vi "EGE_Query.vi"(0 "System no.":i32=1 min=1 max=4 step=1, 2 "Axes to query":string[](array[string]), 3 "All axes?":bool, 4 "Axis identifier?":bool=TRUE, 5 "error in":errorcluster) -> (14 "Electronic gearing mode":bool[](array[boolean]), 19 "error out":errorcluster)   [LabVIEW 2020]
doc: "Returns electronic gearing mode of queried axes.\n\nC-843, C-848, C-880: If All axes = TRUE, then Axis identifier can be FALSE."
panel:
  # "Returns electronic gearing mode for queried axes."
  # "If all axes: use"
  # "Query"
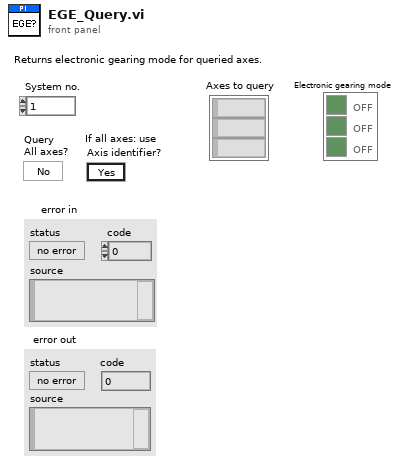
[diagram p1: front panel]
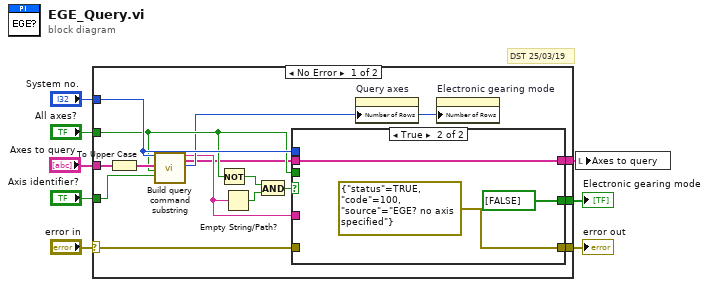
[diagram p0: block diagram]
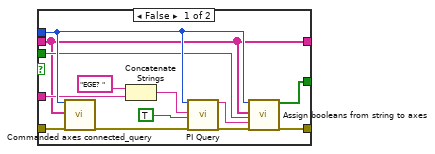
[diagram p2: hidden frame]
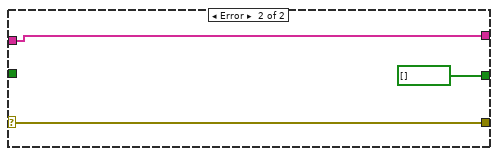
[diagram p3: hidden frame]
diagram:
  # "DST 25/03/19"
  n1 = case shown="No Error" "error in" {
    selector: "error in" -> [w12 w41]
    tunnel: [w23 bool[] [] ("Booleans")] -> w8
    tunnel: "Axes to query" -> [w22 w40]
    tunnel: [w21 w41] -> w6
    tunnel: "Axis identifier?" -> [w19 _]
    tunnel: "System no." -> [w18 _]
    tunnel: [w9 w40] -> w3
    tunnel: "All axes?" -> [w17 _]
    frame No Error {
      n2 = To Upper Case(1:w22) -> (0:w20:string[])
      n3 = call "Build query command substring.vi"("System no."=w18, "Axes to query in"=w20, "Query\nAll axes?"=w17, "For all axes: use\nAxis identifier?"=w19) -> ("Command substring"=w14:string, "Axes to query out"=w10:string[], "Number of rows"=w15:u32)  [unwired: 2 in, 11 out]
      n4 = Not(x=w17) -> (.not. x?=w16:bool)
      n5 = Empty String/Path?(string/path=w14) -> (empty?=w13:bool)
      n6 = And(x=w16, y=w13) -> (x .and. y?=w11:bool)
      n7 = case shown="True" w11 {
        tunnel: [w33 bool[] [FALSE] ("Booleans")] -> w23
        tunnel: [w30 errorcluster {"status"=TRUE, "code"=100, "source"="EGE? no axis specified"} ("error out")] -> w21
        tunnel: w18 -> [w32 _]
        tunnel: w10 -> [w24 w37]
        tunnel: w17 -> [w31 _]
        tunnel: w14 -> [w26 _]
        tunnel: w12 -> [w25 _]
        tunnel: [w24 w37] -> w9
        frame False {
          n8 = call "Commanded axes connected_query.vi"("System no."=w32, "Commanded axes"=w24, "error in"=w25) -> ("error out"=w29:errorcluster)  [unwired: 1 in, 15 out]
          n9 = Concatenate Strings("EGE? ", w26) -> (w34:string)
          n10 = call "PI Query.vi"("System no."=w32, "String to send"=w34, "Attach termination char.?"=TRUE ("Attach Linefeed?"), "error in"=w29) -> ("String read"=w28:string, "error out"=w27:errorcluster)  [unwired: 3 in, 11 out]
          n11 = call "Assign booleans from string to axes.vi"("System no."=w32, "Queried axes"=w24, "All axes queried?"=w31, "Input String"=w28, "error in"=w27) -> ("Booleans"=w33:bool[], "error out"=w30:errorcluster)  [unwired: 13 out]
        }
        frame True {
        }
      }
      n12 = property on="Query axes" class="Arr (strict)"("Number of Rows"=w15) -> ()  [unwired: 2 in, 2 out]
      n13 = property on="Electronic gearing mode" class="Arr (strict)"("Number of Rows"=w15) -> ()  [unwired: 2 in, 2 out]
    }
    frame Error {
    }
  }
  "error out" <- w6
  "Electronic gearing mode" <- w8
  n14 = local write "Axes to query"(w3) -> ()
